vi "ReadATEQData.vi"(11 "Chaîne":string) -> (0 "Prg number":string, 1 "Valeur":i32, 2 "result":string, 3 "Status":string)   [LabVIEW 2020]
uses:
  <vilib>/regexp/Match Regular Expression.xnode
panel:
  out "x != y?":bool
  # "<20>:(AL):PRESSION HAUTE\n<30>:(DR):-126 Pa\n<30>:(DT):2 Pa\n<30>:(DR):-10 Pa\n<30>:(PB):1 Pa\n<30>:(PB):1 Pa\n<30>:(PB):-2 Pa\n<30>:(DR):-197 Pa\n^C"
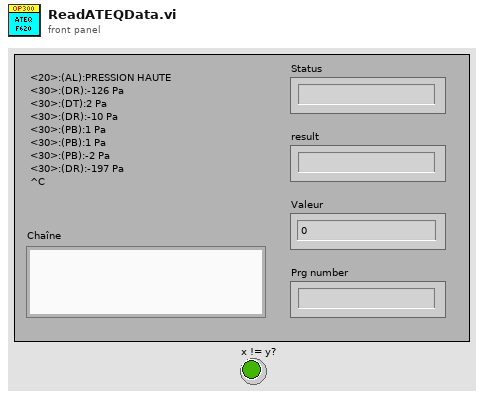
[diagram p1: front panel]
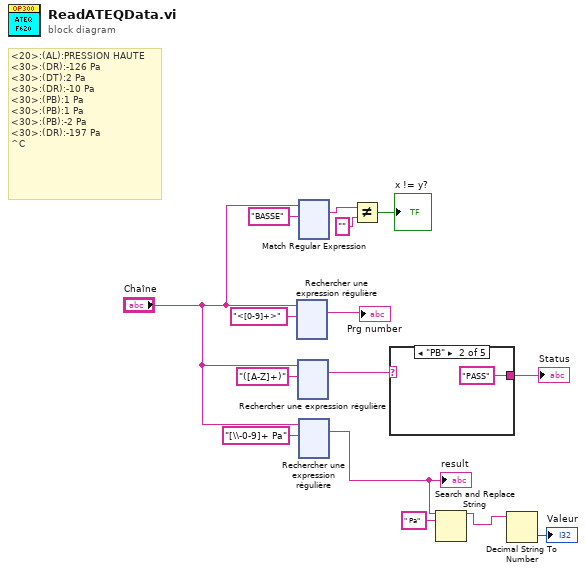
[diagram p0: block diagram]
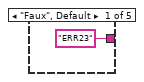
[diagram p2: hidden frame]
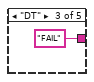
[diagram p3: hidden frame]
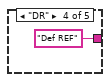
[diagram p4: hidden frame]
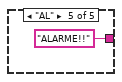
[diagram p5: hidden frame]
diagram:
  # "<20>:(AL):PRESSION HAUTE\n<30>:(DR):-126 Pa\n<30>:(DT):2 Pa\n<30>:(DR):-10 Pa\n<30>:(PB):1 Pa\n<30>:(PB):1 Pa\n<30>:(PB):-2 Pa\n<30>:(DR):-197 Pa\n^C"
  n1 = xnode "Rechercher une expression régulière"("chaîne en entrée"="Chaîne", "expression régulière"="<[0-9]+>") -> ("toute l'expression"=→"Prg number":string)  [unwired: 4 in, 4 out]
  n2 = xnode "Rechercher une expression régulière"("chaîne en entrée"="Chaîne", "expression régulière"="([A-Z]+)") -> ("toute l'expression"=w12:string)  [unwired: 4 in, 4 out]
  n3 = xnode "Match Regular Expression"("input string"="Chaîne", "regular expression"="BASSE") -> ("whole match"=w3:string)  [unwired: 4 in, 4 out]
  n4 = xnode "Rechercher une expression régulière"("chaîne en entrée"="Chaîne", "expression régulière"="[\\-0-9]+ Pa") -> ("toute l'expression"=w9:string)  [unwired: 4 in, 4 out]
  "result" <- w9
  n5 = Not Equal?(x=w3, y="") -> (x != y?=→"x != y?":bool)
  n6 = case shown="\"PB\"" w12 {
    tunnel: ["ERR23" "PASS" "FAIL" "Def REF" "ALARME!!"] -> w11
    frame "Faux", Default {
    }
    frame "PB" {
    }
    frame "DT" {
    }
    frame "DR" {
    }
    frame "AL" {
    }
  }
  "Status" <- w11
  n7 = Search and Replace String ("Rechercher et remplacer une chaîne")(input string=w9, search string=" Pa" ("chaîne recherchée")) -> (result string=w7:string)  [unwired: 6 in, 3 out]
  n8 = Decimal String To Number ("Chaîne décimale en nombre")(string=w7) -> (number=→"Valeur":i32)  [unwired: 2 in, 1 out]
